vi "Event Tree.vi"(8 "error in (no error)":errorcluster, 10 "item":string, 11 "[V] Sys Cfg Main in":refnum<class "[V] Sys Cfg Main.lvclass">) -> (0 "error out":errorcluster, 3 "[V] Sys Cfg Main out":refnum<class "[V] Sys Cfg Main.lvclass">)   [LabVIEW 2020, in "[V] Sys Cfg Main.lvlib" / "[V] Sys Cfg Main.lvclass"]
uses:
  [V] Sys Cfg Main.lvclass
  [V] Sys Cfg Main.lvclass/[V] Sys Cfg Main.ctl
  [V] Sys Cfg Base/[V] Sys Cfg Base Messages/Load Sub Panel Msg/Load Sub Panel Msg.lvclass/Load Sub Panel Msg.ctl
  <vilib>/ActorFramework/Message Enqueuer/Message Enqueuer.lvclass/Message Enqueuer.ctl
  <vilib>/ActorFramework/Message Enqueuer/Enqueue.vi
  [V] Sys Cfg Base/[V] Sys Cfg Base Messages/Load Sub Panel Msg/Load Sub Panel Msg.lvclass
  C:/Program Files (x86)/National Instruments/LabVIEW 2020/vi.lib/ActorFramework/Message/Message.lvclass
  <vilib>/ActorFramework/Message Priority Queue/Priority Enqueue.vi
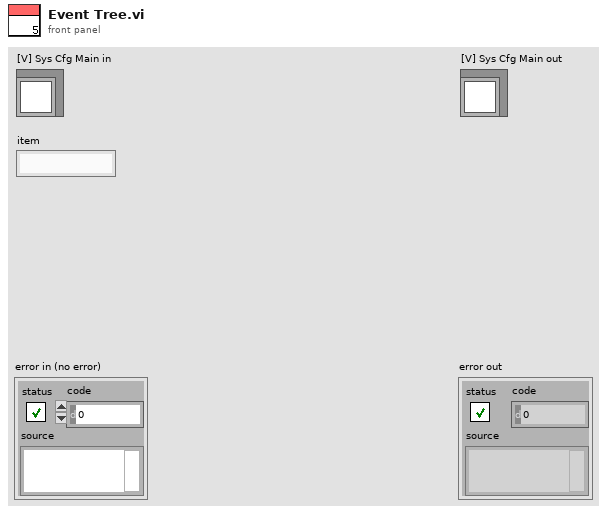
[diagram p1: front panel]
types:
  T1 = map{string, refnum<class "Message Enqueuer.lvclass">}
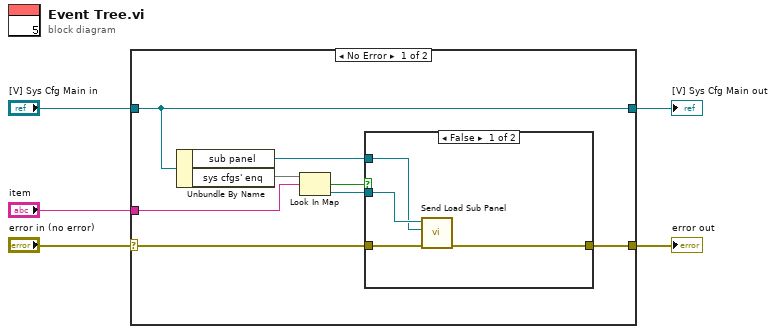
[diagram p0: block diagram]
diagram:
  n1 = case shown="No Error" "error in (no error)" {
    selector: "error in (no error)" -> [w8 w20]
    tunnel: [w6 w20] -> w4
    tunnel: [w13 w19] -> w2
    tunnel: "[V] Sys Cfg Main in" -> [w13 w19]
    tunnel: "item" -> [w9 _]
    frame No Error {
      n2 = Unbundle By Name(w13) -> ("sub panel"=w7:refnum<vi>, "sys cfgs' enq"=w12:T1)
      n3 = Look In Map(map=w12, key=w9) -> (key not found?=w11:bool, value=w10:refnum<class "Message Enqueuer.lvclass">)  [unwired: 1 in]
      n4 = case shown="False" w11 {
        tunnel: w10 -> [w16 _]
        tunnel: w8 -> [w17 w18]
        tunnel: w7 -> [w15 _]
        tunnel: [w14 w18] -> w6
        frame False {
          n5 = call "Send Load Sub Panel.vi"("error in (no error)"=w17, "sub panel ref"=w15, "Message Enqueuer"=w16) -> ("error out"=w14:errorcluster)  [unwired: 7 in, 1 out]
        }
        frame True {
        }
      }
    }
    frame Error {
    }
  }
  "error out" <- w4
  "[V] Sys Cfg Main out" <- w2
